vi "Destroy.vi"(0 "reference in":refnum<class "SmartMotor.lvclass">, 5 "error in (no error)":errorcluster) -> (14 "reference out":refnum<class "SmartMotor.lvclass">, 19 "error out":errorcluster)   [LabVIEW 2017, in "SmartMotor.lvclass"]
uses:
  SmartMotor.lvclass
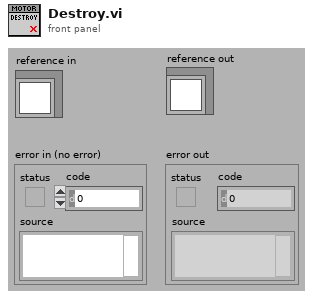
[diagram p1: front panel]
types:
  T1 = typedef "SmartMotor.lvclass/ObjectAttributes.ctl" = cluster{"SmartMotor Chain VISA Resource":refnum<visa-resource-name>, "SmartMotor Chain Address":i16, "Motor Absolute Position":i32, "Motor Relative Position":i32, "Motor Torque":i32, "Motor Voltage":i32, "Screwdriver Engaged":bool, "Screwdriver Torque Limit":i32, "Torque Monitor On/Off Status":bool, "Torque Monitor VI Reference":refnum<vi>, "Absolute Motor Torque (Filtered)":dbl, "SmartMotor Status":T2, "SmartMotor Error":T3}
  T2 = typedef "SmartMotor.lvclass/SmartMotor Status.ctl" = enum8{"Stopped", "Moving"}
  T3 = typedef "SmartMotor.lvclass/SmartMotor Error.ctl" = enum8{"None", "Read Error", "Low Voltage"}
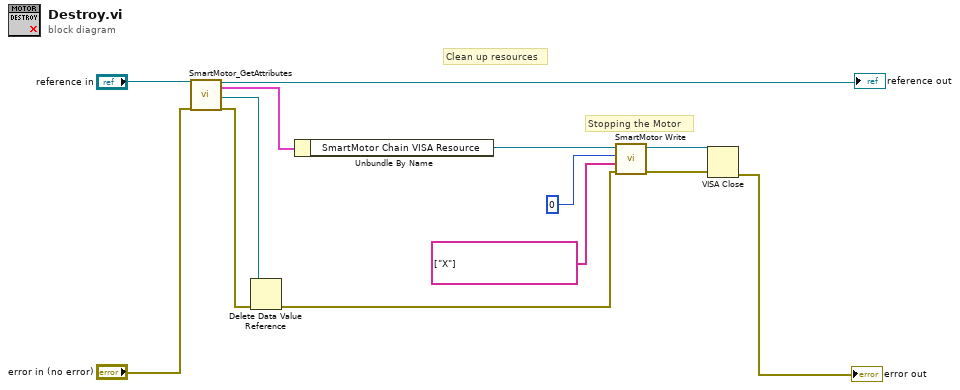
[diagram p0: block diagram]
diagram:
  # "Stopping the Motor"
  # "Clean up resources"
  n1 = call "SmartMotor_GetAttributes.vi"("reference in"="reference in", "error in (no error)"="error in (no error)") -> ("reference out"=→"reference out":refnum<class "SmartMotor.lvclass">, "Data"=w9:T1, "DataRef"=w10:refnum<data-value>, "error out"=w11:errorcluster)  [unwired: 14 in]
  n2 = Delete Data Value Reference(data value reference=w10, error in=w11) -> (error out=w4:errorcluster)  [unwired: 1 out]
  n3 = Unbundle By Name(w9) -> ("SmartMotor Chain VISA Resource"=w8:refnum<visa-resource-name>)
  n4 = call "SmartMotor Write.vi"("VISA resource IN"=w8, "Motor Number"=u8 0, "Motor Command Array"=string[] ["X"], "Error In"=w4) -> ("VISA resource OUT"=w1:refnum<visa-resource-name>, "Error Out"=w3:errorcluster)  [unwired: 3 in, 1 out]
  n5 = VISA Close(VISA resource name=w1, error in (no error)=w3) -> (error out=→"error out":errorcluster)
